vi "Main.vi"() -> ()   [LabVIEW 2020]
uses:
  Gamepad_Interface.ctl
  <vilib>/High Genius/HG_WSI_Tookit/Dependencies/Library/CAN/CAN.lvclass
  C:/Program Files (x86)/National Instruments/LabVIEW 2020/vi.lib/High Genius/HG_WSI_Tookit/Dependencies/Library/HG_LIB/HG_LIB.lvclass
  <vilib>/High Genius/HG_WSI_Tookit/Dependencies/Library/PWM/PWM.lvclass
  <vilib>/Platform/TimedLoop/XDataNode/timing_clust.ctl
  <vilib>/Platform/TimedLoop/XDataNode/nitl_modes.ctl
  <vilib>/Platform/TimedLoop/XDataNode/wakeup.ctl
  <vilib>/Platform/TimedLoop/XDataNode/XDataNode.xnode
  <vilib>/Platform/TimedLoop/XDataNode/XDNodeRunTimeDep.lvlib
  <vilib>/High Genius/HG_WSI_Tookit/Dependencies/Library/HG_LIB/HG_LIB.lvclass
panel:
  out "Boolean 2":bool
  out "Boolean":bool
  out "B":bool
  out "X":bool
  in  "PD2":dbl
  in  "PD1":dbl
  out "Numeric":dbl
  out "error out 3":errorcluster
  out "error out 2":errorcluster
  in  "R":dbl min=-255.0 max=255.0 step=1.0
  in  "L":dbl min=-255.0 max=255.0 step=1.0
  in  "B":dbl min=-255.0 max=255.0 step=1.0
  out "error out":errorcluster
  out "type":T1 {"RStick_Y" scale=-1.0..1.0; "RStick_X" scale=-1.0..1.0; "LStick_Y" scale=-1.0..1.0; "RStick_X" scale=-1.0..1.0; "RT" scale=-1.0..1.0; "LT" scale=-1.0..1.0}
  in  "stop":bool
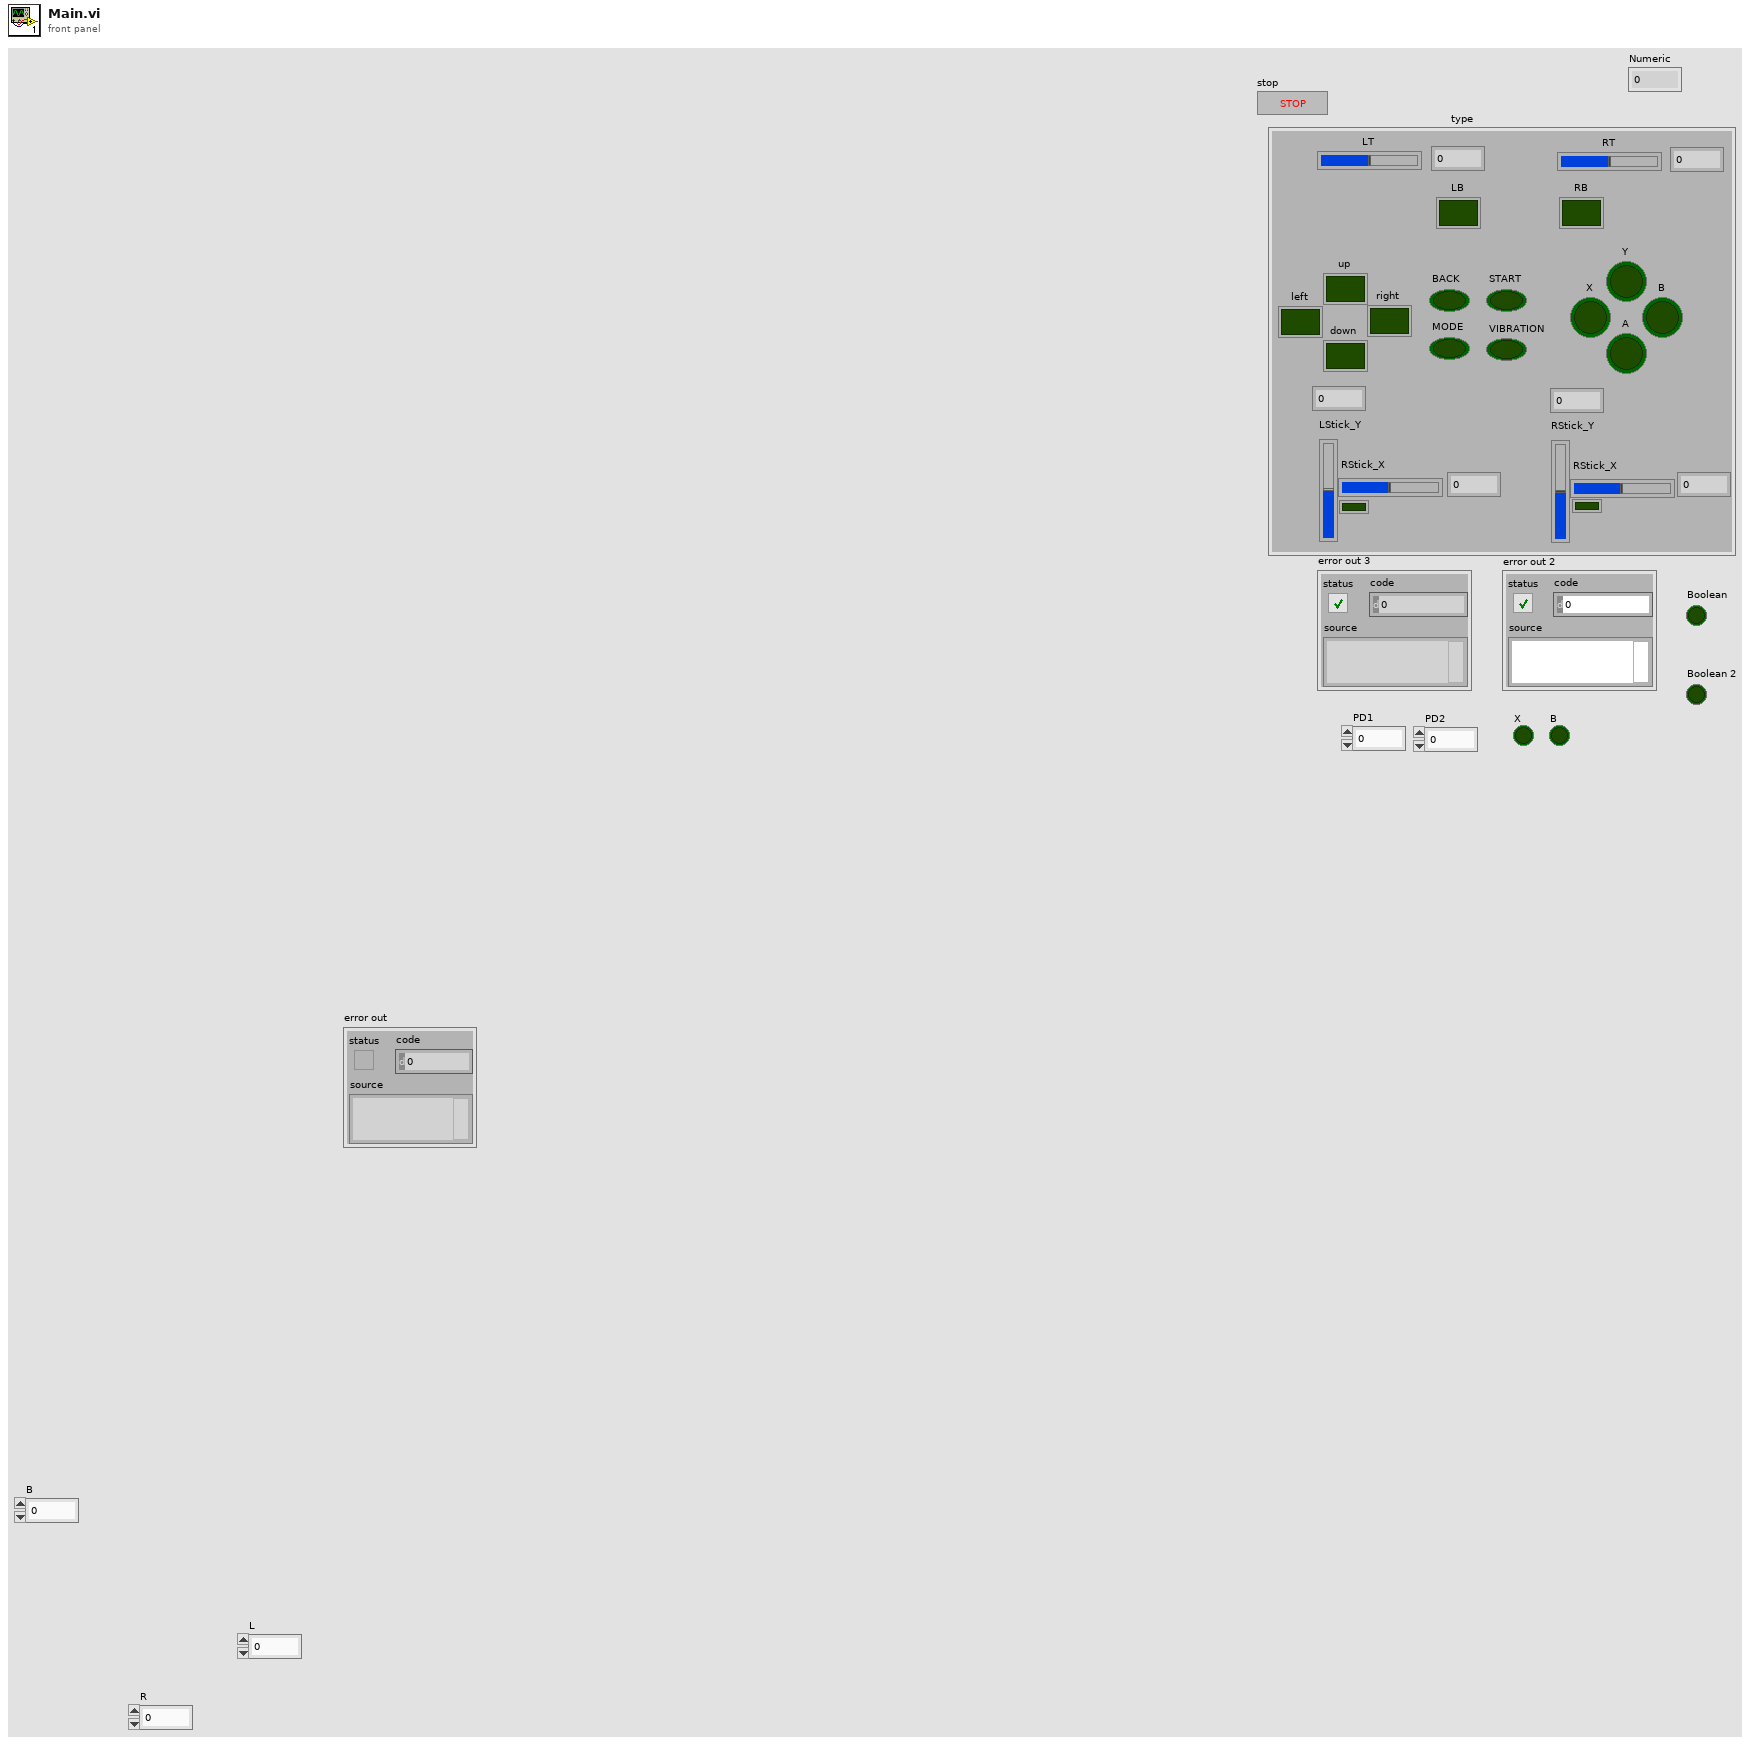
[diagram p1: front panel]
types:
  T1 = typedef "Gamepad_Interface.ctl" = cluster{"left":bool, "up":bool, "down":bool, "right":bool, "Y":bool, "X":bool, "A":bool, "B":bool, "BACK":bool, "START":bool, "MODE":bool, "VIBRATION":bool, "LB":bool, "RB":bool, "LT":dbl, "RT":dbl, "RStick_X":dbl, "LStick_Y":dbl, "RStick_X":dbl, "RStick_Y":dbl, "左杆":bool, "右杆":bool}
  T2 = enum16{"DI", "DO", "AI", "Pulse", "PWM", "ISQ", "ENC", "CAN", "IIC", "IMU"}
  T3 = enum16{"0", "1", "2", "3", "4", "5", "6", "7", "8", "9", "10", "11", "12", "13", "14", "15", "16", "17", "18", "19", "20", "21", "22", "23", "24", "25"}
  T4 = typedef "XDNodeRunTimeDep.lvlib/timing_clust.ctl" = cluster{"Expected End [f-1]":u64, "Actual End [f-1]":u64, "Finished Late? [f-1]":bool, "Expected End [i-1]":u64, "Actual End [i-1]":u64, "Finished Late? [i-1]":bool, "Expected Start [i]":u64, "Actual Start [i]":u64, "Expected Start [f]":u64, "Actual Start [f]":u64, "Source Name":string, "Structure Name":string, "Period":i64, "Deadline":i64, "Offset":i64, "Start":i64, "Priority":i32, "Timeout":i32, "Mode":T5, "Wakeup Reason":T6, "Error":errorcluster, "Source Type":string, "Secondary Source Type":string, "Global End Time":u64, "Global Start Time":u64, "Frame Duration":u64, "Iteration Duration":u64, "Assigned CPU":i32, "I/O Scan Engine Mode":u32}
  T5 = typedef "XDNodeRunTimeDep.lvlib/nitl_modes.ctl" = enum32{"No Change", "Process missed periods, maintain original phase", "Discard missed periods, maintain original phase", "Process missed periods, ignore original phase", "Discard missed periods, ignore original phase"}
  T6 = typedef "XDNodeRunTimeDep.lvlib/wakeup.ctl" = enum32{"Normal", "Aborted", "Asynchronous wakeup", "Timing source error", "Timed loop error", "Timeout"}
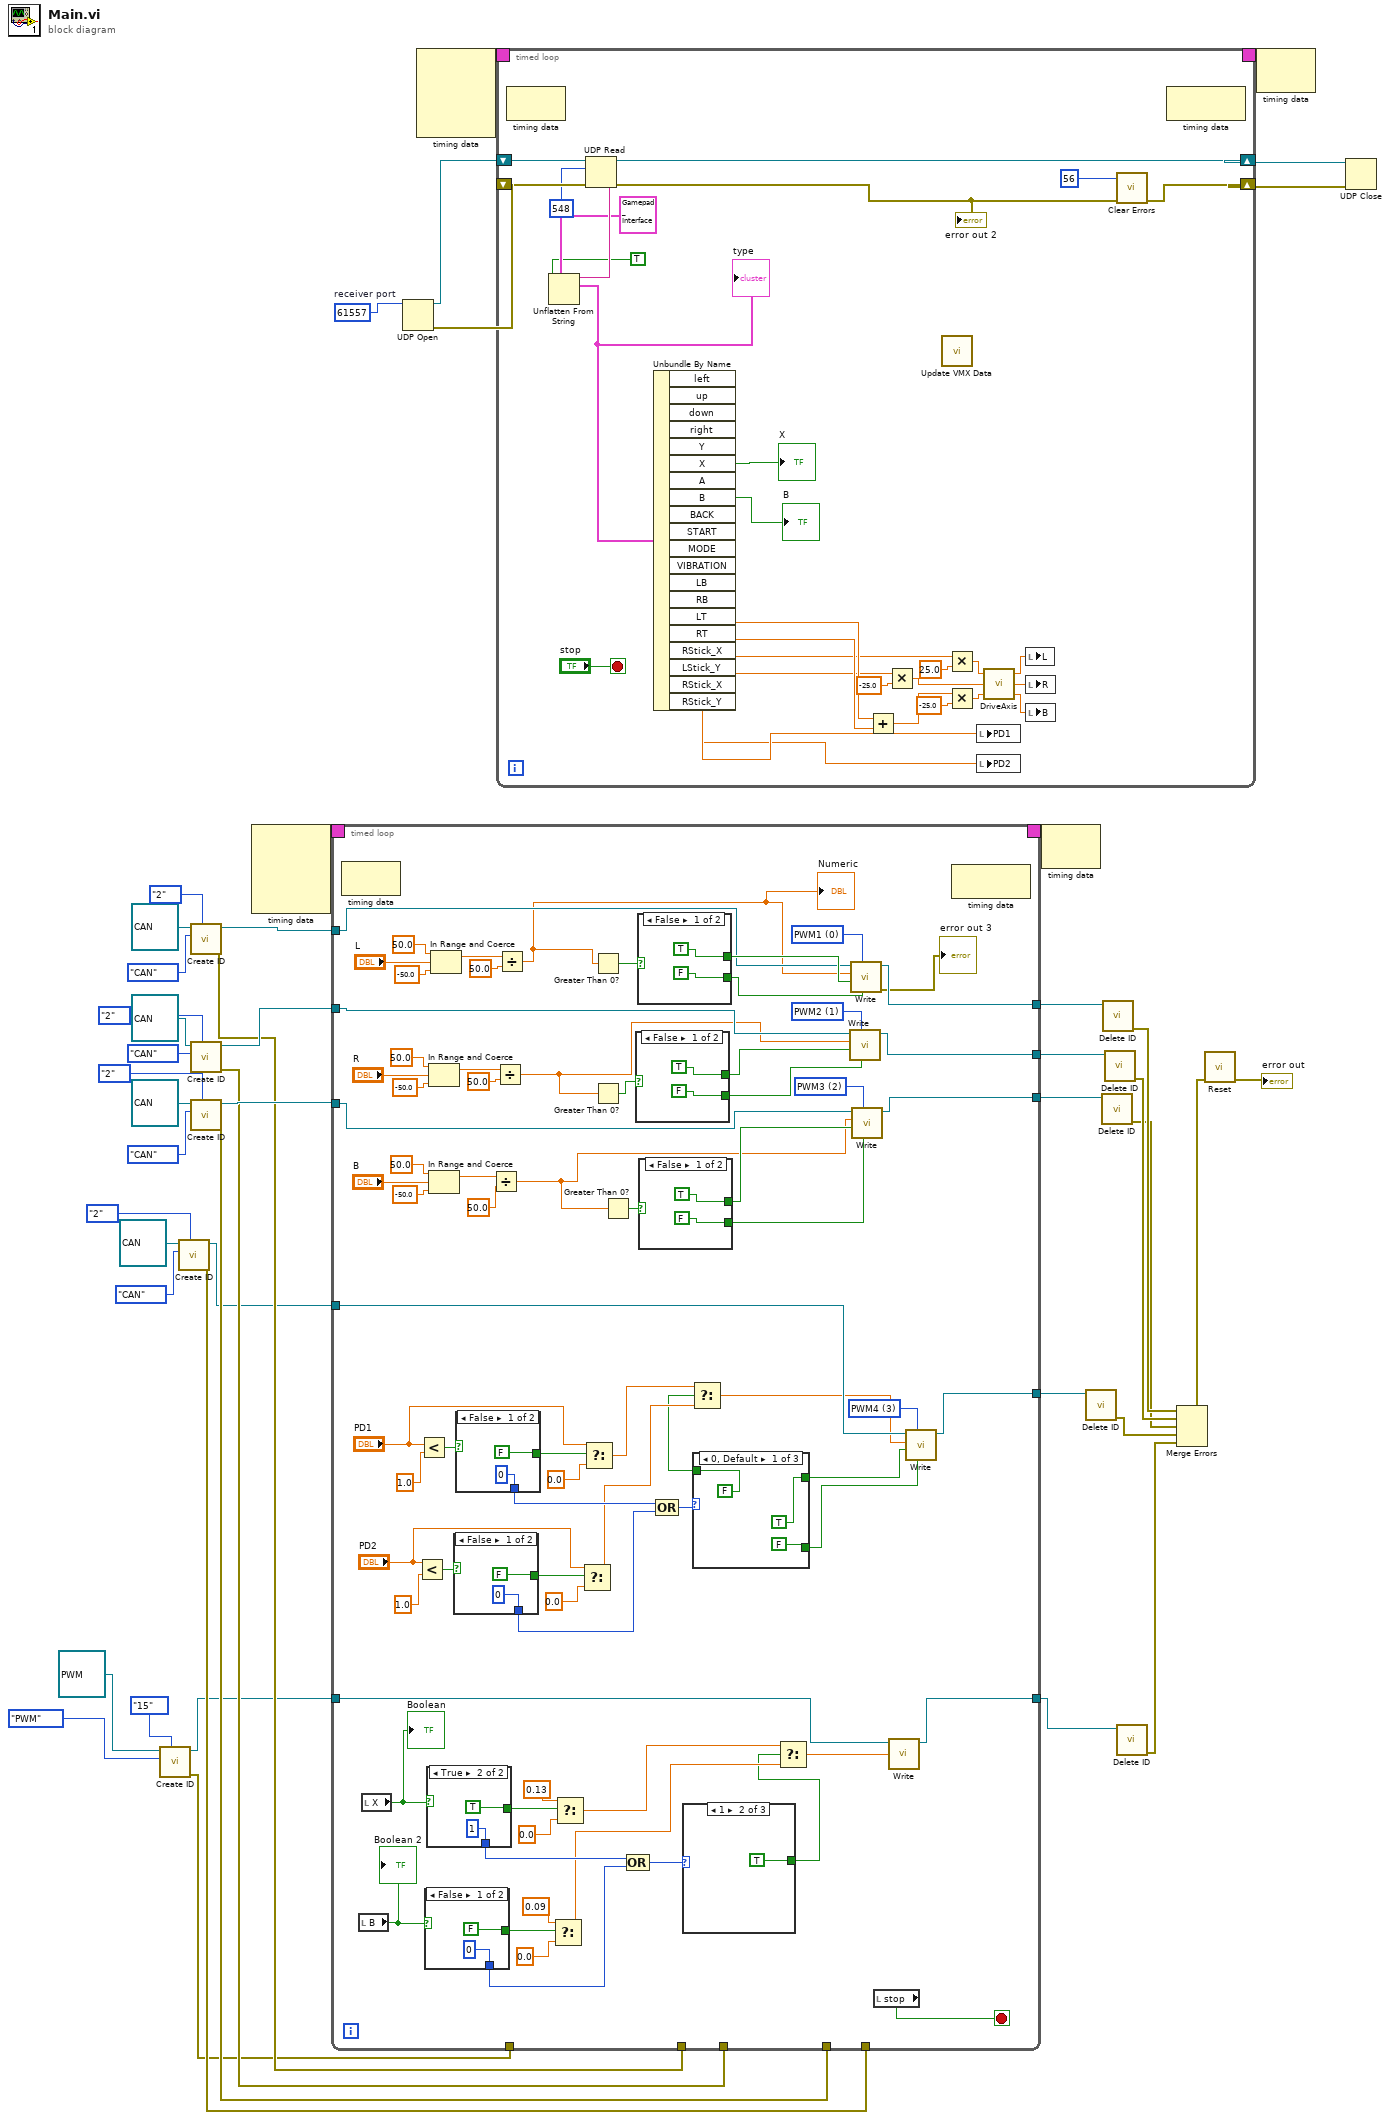
[diagram p0: block diagram]
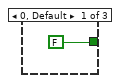
[diagram p2: hidden frame]
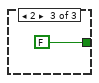
[diagram p3: hidden frame]
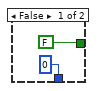
[diagram p4: hidden frame]
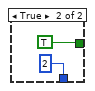
[diagram p5: hidden frame]
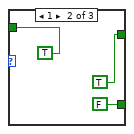
[diagram p6: hidden frame]
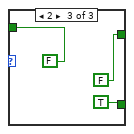
[diagram p7: hidden frame]
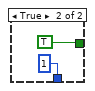
[diagram p8: hidden frame]
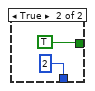
[diagram p9: hidden frame]
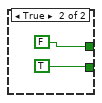
[diagram p10: hidden frame]
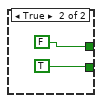
[diagram p11: hidden frame]
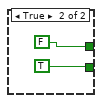
[diagram p12: hidden frame]
diagram:
  w42 = u16 61557  # receiver port
  n1 = call <vilib>:"Create ID.vi"("NO"=T3."15", "Function"=T2."PWM", "HG_LIB in"=refnum<class "PWM.lvclass"> refnum ("VMX Library.lvlib:PWM.lvclass")) -> ("error out"=w1:errorcluster, "HG_LIB out"=w2:refnum<class "PWM.lvclass">)  [unwired: 7 in]
  n2 = call <vilib>:"Create ID.vi"("NO"=T3."2", "Function"=T2."CAN", "HG_LIB in"=refnum<class "CAN.lvclass"> refnum ("VMX Library.lvlib:CAN.lvclass")) -> ("error out"=w10:errorcluster, "HG_LIB out"=w11:refnum<class "CAN.lvclass">)  [unwired: 7 in]
  n3 = call <vilib>:"Create ID.vi"("NO"=T3."2", "Function"=T2."CAN", "HG_LIB in"=refnum<class "CAN.lvclass"> refnum ("VMX Library.lvlib:CAN.lvclass")) -> ("error out"=w27:errorcluster, "HG_LIB out"=w31:refnum<class "CAN.lvclass">)  [unwired: 7 in]
  n4 = call <vilib>:"Create ID.vi"("NO"=T3."2", "Function"=T2."CAN", "HG_LIB in"=refnum<class "CAN.lvclass"> refnum ("VMX Library.lvlib:CAN.lvclass")) -> ("error out"=w26:errorcluster, "HG_LIB out"=w30:refnum<class "CAN.lvclass">)  [unwired: 7 in]
  n5 = call <vilib>:"Create ID.vi"("NO"=T3."2", "Function"=T2."CAN", "HG_LIB in"=refnum<class "CAN.lvclass"> refnum ("VMX Library.lvlib:CAN.lvclass")) -> ("error out"=w25:errorcluster, "HG_LIB out"=w29:refnum<class "CAN.lvclass">)  [unwired: 7 in]
  n6 = node-c288() -> (w39:T4)  [unwired: 4 in]
  n7 = timed-loop {
    timing: w39 -> [_]
    timing-out: [_] -> w38
    tunnel: w29 -> [w93]
    tunnel: w30 -> [w94]
    tunnel: w31 -> [w95]
    tunnel: w27 -> [_]
    tunnel: w26 -> [_]
    tunnel: w25 -> [_]
    tunnel: [w98] -> w20
    tunnel: [w97] -> w19
    tunnel: [w96] -> w18
    tunnel: w11 -> [w84]
    tunnel: w10 -> [_]
    tunnel: [w64] -> w6
    tunnel: w1 -> [_]
    tunnel: w2 -> [w62]
    tunnel: [w63] -> w4
    stop <- w123 stop-if-true
    w85 = u16 3 items=["PWM1", "PWM2", "PWM3", "PWM4"] ("PWM")
    w106 = u16 1 items=["PWM1", "PWM2", "PWM3", "PWM4"] ("PWM")
    w105 = u16 0 items=["PWM1", "PWM2", "PWM3", "PWM4"] ("PWM")
    w121 = u16 2 items=["PWM1", "PWM2", "PWM3", "PWM4"] ("PWM")
    n8 = node-c288() -> ()  [unwired: 1 in, 1 out]
    n9 = local read "B"() -> (w50:bool)
    "Boolean 2" <- w50
    n10 = local read "X"() -> (w51:bool)
    "Boolean" <- w51
    n11 = Less?(x="PD2", y=1.0) -> (x < y?=w82:bool)
    n12 = Less?(x="PD1", y=1.0) -> (x < y?=w77:bool)
    n13 = case shown="False" w50 {
      tunnel: [FALSE TRUE] -> w61
      tunnel: [0 2] -> w56
      frame False {
      }
      frame True {
      }
    }
    n14 = case shown="True" w51 {
      tunnel: [FALSE TRUE] -> w59
      tunnel: [0 1] -> w57
      frame False {
      }
      frame True {
      }
    }
    n15 = In Range and Coerce(upper limit=50.0, x="R", lower limit=-50.0 ("upper limit")) -> (coerced(x)=w120:dbl)  [unwired: 1 out]
    n16 = In Range and Coerce(upper limit=50.0, x="B", lower limit=-50.0 ("upper limit")) -> (coerced(x)=w110:dbl)  [unwired: 1 out]
    n17 = In Range and Coerce(upper limit=50.0, x="L", lower limit=-50.0 ("upper limit")) -> (coerced(x)=w113:dbl)  [unwired: 1 out]
    n18 = case shown="False" w82 {
      tunnel: [FALSE TRUE] -> w80
      tunnel: [0 2] -> w72
      frame False {
      }
      frame True {
      }
    }
    n19 = case shown="False" w77 {
      tunnel: [FALSE TRUE] -> w75
      tunnel: [0 1] -> w73
      frame False {
      }
      frame True {
      }
    }
    n20 = Divide(x=w110, y=50.0 ("x")) -> (x/y=w91:dbl)
    n21 = Divide(x=w120, y=50.0 ("x")) -> (x/y=w88:dbl)
    n22 = Divide(x=w113, y=50.0 ("x")) -> (x/y=w86:dbl)
    "Numeric" <- w86
    n23 = Select(t=0.09, s=w61, f=0.0) -> (s? t:f=w54:dbl)
    n24 = Select(t=0.13, s=w59, f=0.0) -> (s? t:f=w55:dbl)
    n25 = Select(t="PD2", s=w80, f=0.0) -> (s? t:f=w67:dbl)
    n26 = Select(t="PD1", s=w75, f=0.0) -> (s? t:f=w68:dbl)
    n27 = Greater Than 0?(x=w86) -> (x > 0?=w90:bool)
    n28 = Greater Than 0?(x=w88) -> (x > 0?=w89:bool)
    n29 = Greater Than 0?(x=w91) -> (x > 0?=w92:bool)
    n30 = Compound Arithmetic op=OR(w57, w56) -> (w49:i32)
    n31 = case shown="False" w89 {
      tunnel: [TRUE FALSE] -> w102
      tunnel: [FALSE TRUE] -> w101
      frame False {
      }
      frame True {
      }
    }
    n32 = case shown="False" w90 {
      tunnel: [TRUE FALSE] -> w104
      tunnel: [FALSE TRUE] -> w103
      frame False {
      }
      frame True {
      }
    }
    n33 = case shown="False" w92 {
      tunnel: [TRUE FALSE] -> w100
      tunnel: [FALSE TRUE] -> w99
      frame False {
      }
      frame True {
      }
    }
    n34 = Compound Arithmetic op=OR(w73, w72) -> (w71:i32)
    n35 = case shown="1" w49 {
      tunnel: [FALSE TRUE FALSE] -> w48
      frame 0, Default {
      }
      frame 1 {
      }
      frame 2 {
      }
    }
    n36 = case shown="0, Default" w71 {
      tunnel: [TRUE TRUE FALSE] -> w70
      tunnel: [FALSE FALSE TRUE] -> w69
      tunnel: [FALSE TRUE FALSE] -> w66
      frame 0, Default {
      }
      frame 1 {
      }
      frame 2 {
      }
    }
    n37 = Select(t=w68, s=w66, f=w67) -> (s? t:f=w83:dbl)
    n38 = Select(t=w55, s=w48, f=w54) -> (s? t:f=w47:dbl)
    n39 = call <vilib>:"Write.vi"("INB"=w101, "PWM"=w106, "INA"=w102, "Duty Cycle"=w88, "CAN in"=w94) -> ("CAN out"=w97:refnum<class "CAN.lvclass">)  [unwired: 5 in, 1 out]
    n40 = call <vilib>:"Write.vi"("INB"=w103, "PWM"=w105, "INA"=w104, "Duty Cycle"=w86, "CAN in"=w95) -> ("error out"=→"error out 3":errorcluster, "CAN out"=w98:refnum<class "CAN.lvclass">)  [unwired: 5 in]
    n41 = call <vilib>:"Write.vi"("INB"=w99, "PWM"=w121, "INA"=w100, "Duty Cycle"=w91, "CAN in"=w93) -> ("CAN out"=w96:refnum<class "CAN.lvclass">)  [unwired: 5 in, 1 out]
    n42 = local read "stop"() -> (w123:bool)
    n43 = call <vilib>:"Write.vi"("PWM"=w47, "PWM in"=w62) -> ("PWM out"=w63:refnum<class "PWM.lvclass">)  [unwired: 8 in, 1 out]
    n44 = call <vilib>:"Write.vi"("INB"=w69, "PWM"=w85, "INA"=w70, "Duty Cycle"=w83, "CAN in"=w84) -> ("CAN out"=w64:refnum<class "CAN.lvclass">)  [unwired: 5 in, 1 out]
    n45 = node-c288() -> ()  [unwired: 1 in, 1 out]
  }
  n46 = UDP Open(11:w42) -> (port=w41:refnum<k16>, 0:w40:errorcluster)  [unwired: 4 in, 1 out]
  n47 = node-c288() -> (w46:T4)  [unwired: 4 in]
  n48 = timed-loop {
    timing: w46 -> [_]
    timing-out: [_] -> w45
    shift-right: [w193] -> w44
    shift-left: w41 -> [w195]
    shift-right: [w191] -> w43
    shift-left: w40 -> [w194]
    stop <- "stop" stop-if-true
    n49 = node-c288() -> ()  [unwired: 1 in, 1 out]
    n50 = UDP Read(connection ID=w195, max size (548)=548, 8:w194) -> (data out=w190:string, error out=w192:errorcluster, 3:w193:refnum<k16>)  [unwired: 1 in, 2 out]
    "error out 2" <- w192
    n51 = Unflatten From String(type=T1 {"left"=FALSE, "up"=FALSE, "down"=FALSE, "right"=FALSE, "Y"=FALSE, "X"=FALSE, "A"=FALSE, "B"=FALSE, "BACK"=FALSE, "START"=FALSE, "MODE"=FALSE, "VIBRATION"=FALSE, "LB"=FALSE, "RB"=FALSE, "LT"=0.0, "RT"=0.0, "RStick_X"=0.0, "LStick_Y"=0.0, "RStick_X"=0.0, "RStick_Y"=0.0, "左杆"=FALSE, "右杆"=FALSE} ("Gamepad_Interface"), binary string=w190, data includes array or string size? (T)=TRUE) -> (value=w186:T1)  [unwired: 2 in, 2 out]
    "type" <- w186
    n52 = Unbundle By Name(w186) -> ("X"=→"X":bool, "B"=→"B":bool, "LT"=w185:dbl, "RT"=w184:dbl, "RStick_X"=w181:dbl, "LStick_Y"=w180:dbl, "RStick_X"=w168:dbl, "RStick_Y"=w169:dbl)  [unwired: 12 out]
    n53 = Add(x=w185, y=w184) -> (x+y=w173:dbl)
    n54 = Multiply(x=w180, y=-25.0) -> (x*y=w178:dbl)
    n55 = call <vilib>:"Update VMX Data.vi"() -> ()  [unwired: 11 in, 1 out]
    n56 = Multiply(x=w181, y=25.0) -> (x*y=w179:dbl)
    n57 = Multiply(x=w173, y=-25.0) -> (x*y=w177:dbl)
    n58 = local write "PD1"(w169) -> ()
    n59 = local write "PD2"(w168) -> ()
    n60 = call "DriveAxis.vi"("Theta"=w177, "Y"=w178, "X"=w179) -> ("B"=w174:dbl, "R"=w175:dbl, "L"=w176:dbl)
    n61 = local write "L"(w176) -> ()
    n62 = local write "R"(w175) -> ()
    n63 = local write "B"(w174) -> ()
    n64 = call <vilib>:"Clear Errors.vi"("error in (no error)"=w192, "specific error code to clear (0: all)"=56) -> ("error out"=w191:errorcluster)  [unwired: 4 in, 1 out]
    n65 = node-c288() -> ()  [unwired: 1 in, 1 out]
  }
  n66 = node-c288(w38) -> ()  [unwired: 1 out]
  n67 = call <vilib>:"Delete ID.vi"("HG_LIB in"=w6) -> ("error out"=w5:errorcluster)  [unwired: 9 in, 1 out]
  n68 = call <vilib>:"Delete ID.vi"("HG_LIB in"=w18) -> ("error out"=w22:errorcluster)  [unwired: 9 in, 1 out]
  n69 = call <vilib>:"Delete ID.vi"("HG_LIB in"=w20) -> ("error out"=w24:errorcluster)  [unwired: 9 in, 1 out]
  n70 = call <vilib>:"Delete ID.vi"("HG_LIB in"=w19) -> ("error out"=w23:errorcluster)  [unwired: 9 in, 1 out]
  n71 = call <vilib>:"Delete ID.vi"("HG_LIB in"=w4) -> ("error out"=w3:errorcluster)  [unwired: 9 in, 1 out]
  n72 = Merge Errors(w24, w23, w22, w5, w3) -> (w21:errorcluster)
  n73 = call <vilib>:"Reset.vi"("error in (no error)"=w21) -> ("error out"=→"error out":errorcluster)  [unwired: 10 in]
  n74 = node-c288(w45) -> ()  [unwired: 1 out]
  n75 = UDP Close(connection ID=w44, 8:w43) -> ()  [unwired: 2 out]
